vi "create.from_array_pairs.vi"(10 "Array Pairs":cluster{"name":string[], "value":string[]}) -> (3 "properties out":refnum<class "properties.lvclass">)   [LabVIEW 2020, in "nominal types.lvlib" / "properties.lvclass"]
uses:
  properties.lvclass
  properties.lvclass/properties.ctl
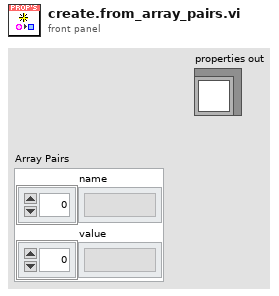
[diagram p1: front panel]
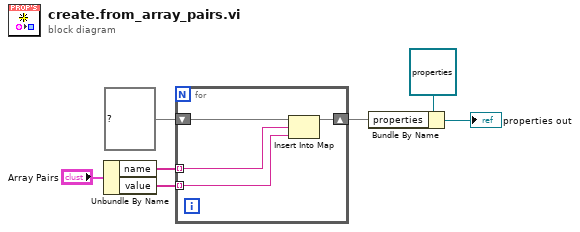
[diagram p0: block diagram]
diagram:
  n1 = Unbundle By Name("Array Pairs") -> ("name"=w2:string[], "value"=w1:string[])
  n2 = for {
    shift-right: [w10] -> w4
    shift-left: map{string, string} {} ("properties") -> [w11]
    tunnel: w2 -> [w9] mode=indexing
    tunnel: w1 -> [w8] mode=indexing
    n3 = Insert Into Map(map in=w11, key=w9, value=w8) -> (map out=w10:map{string, string})  [unwired: 2 out]
  }
  n4 = Bundle By Name(cluster=refnum<class "properties.lvclass"> refnum ("properties out"), "properties"=w4) -> (→"properties out":refnum<class "properties.lvclass">)
